vi "CMC温度读取.vi"(8 "error in":errorcluster caption="错误输入", 11 "Channel":u16=81 format="%.0x") -> (0 "error out":errorcluster caption="错误输出", 2 "CMC1温度":i32[](array[numeric]), 3 "CMC2温度":i32[](array[numeric]))   [LabVIEW 2020]
uses:
  <userlib>/PCANBasic/PCANBasic.lvlib
panel:
  out "function return 2":u32 format="%.0x"
  out "function return 3":u32 format="%.0x"
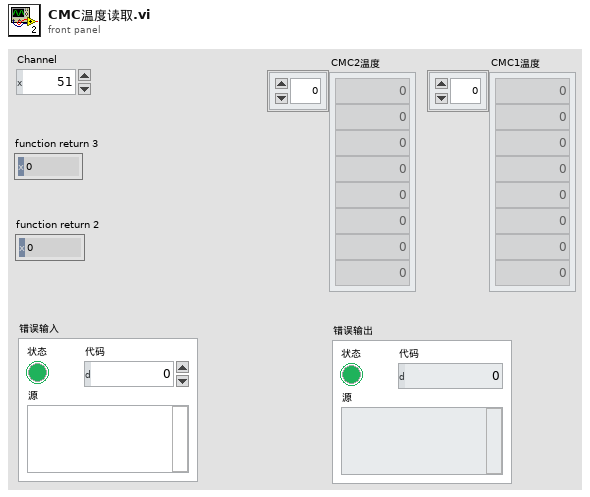
[diagram p1: front panel]
types:
  T1 = typedef "PCANBasic.lvlib/TPCANStatus.ctl" = u32
  T2 = typedef "PCANBasic.lvlib/TPCANMsgFD.ctl" = cluster{"ID":u32, "MSGTYPE":u8, "DLC":u8, "DATA":cluster{"[0]":u8, "[1]":u8, "[2]":u8, "[3]":u8, "[4]":u8, "[5]":u8, "[6]":u8, "[7]":u8, "[8]":u8, "[9]":u8, "[10]":u8, "[11]":u8, "[12]":u8, "[13]":u8, "[14]":u8, "[15]":u8, "[16]":u8, "[17]":u8, "[18]":u8, "[19]":u8, "[20]":u8, "[21]":u8, "[22]":u8, "[23]":u8, "[24]":u8, "[25]":u8, "[26]":u8, "[27]":u8, "[28]":u8, "[29]":u8, "[30]":u8, "[31]":u8, "[32]":u8, "[33]":u8, "[34]":u8, "[35]":u8, "[36]":u8, "[37]":u8, "[38]":u8, "[39]":u8, "[40]":u8, "[41]":u8, "[42]":u8, "[43]":u8, "[44]":u8, "[45]":u8, "[46]":u8, "[47]":u8, "[48]":u8, "[49]":u8, "[50]":u8, "[51]":u8, "[52]":u8, "[53]":u8, "[54]":u8, "[55]":u8, "[56]":u8, "[57]":u8, "[58]":u8, "[59]":u8, "[60]":u8, "[61]":u8, "[62]":u8, "[63]":u8}}
  T3 = cluster{"[0]":u8, "[1]":u8, "[2]":u8, "[3]":u8, "[4]":u8, "[5]":u8, "[6]":u8, "[7]":u8, "[8]":u8, "[9]":u8, "[10]":u8, "[11]":u8, "[12]":u8, "[13]":u8, "[14]":u8, "[15]":u8, "[16]":u8, "[17]":u8, "[18]":u8, "[19]":u8, "[20]":u8, "[21]":u8, "[22]":u8, "[23]":u8, "[24]":u8, "[25]":u8, "[26]":u8, "[27]":u8, "[28]":u8, "[29]":u8, "[30]":u8, "[31]":u8, "[32]":u8, "[33]":u8, "[34]":u8, "[35]":u8, "[36]":u8, "[37]":u8, "[38]":u8, "[39]":u8, "[40]":u8, "[41]":u8, "[42]":u8, "[43]":u8, "[44]":u8, "[45]":u8, "[46]":u8, "[47]":u8, "[48]":u8, "[49]":u8, "[50]":u8, "[51]":u8, "[52]":u8, "[53]":u8, "[54]":u8, "[55]":u8, "[56]":u8, "[57]":u8, "[58]":u8, "[59]":u8, "[60]":u8, "[61]":u8, "[62]":u8, "[63]":u8}
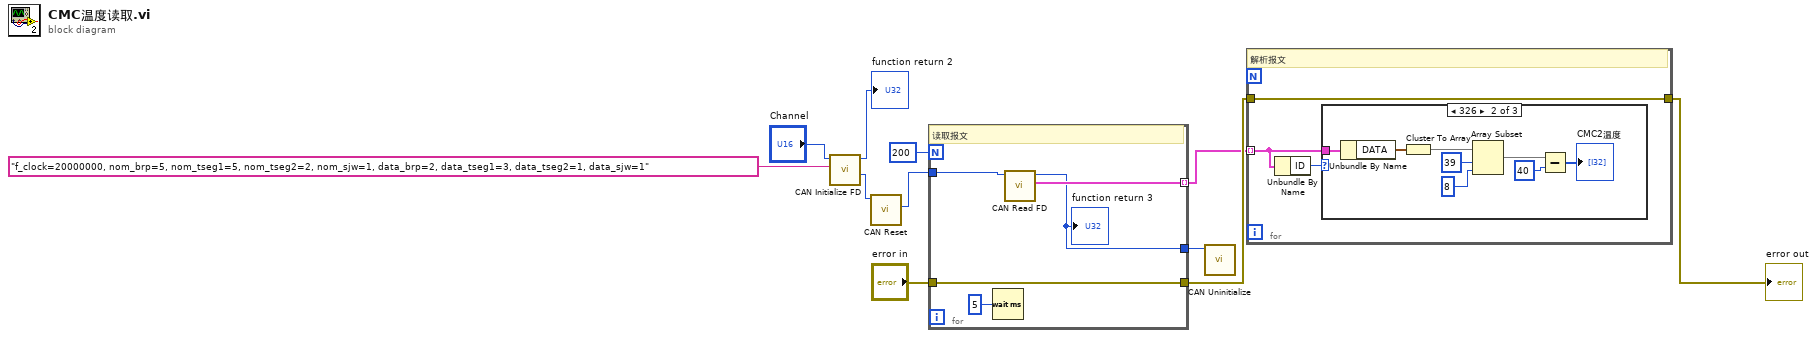
[diagram p0: block diagram]
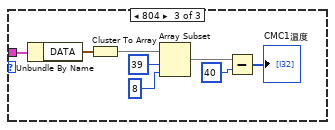
[diagram p3: hidden frame]
diagram:
  n1 = call <userlib>:"CAN Initialize FD.vi"("BitrateFD"="f_clock=20000000, nom_brp=5, nom_tseg1=5, nom_tseg2=2, nom_sjw=1, data_brp=2, data_tseg1=3, data_tseg2=1, data_sjw=1", "Channel"="Channel") -> ("Channel out"=w3:u16, "TCANStatus"=→"function return 2":T1)  [unwired: 6 in, 2 out]
  n2 = call <userlib>:"CAN Reset.vi"("Channel in"=w3) -> ("Channel out"=w2:u16)  [unwired: 8 in, 2 out]
  n3 = for {
    N: 200 -> [_]
    tunnel: [w15] -> w1 mode=indexing
    tunnel: [w14] -> w7
    tunnel: "error in" -> [w13]
    tunnel: [w13] -> w5
    tunnel: w2 -> [w12]
    # "读取报文"
    n4 = Wait (ms)(milliseconds to wait=u32 5 ("等待时间（毫秒）")) -> ()  [unwired: 1 out]
    n5 = call <userlib>:"CAN Read FD.vi"("Channel"=w12) -> ("MessageBuffer out"=w15:T2, "TCANStatus"=w14:T1)  [unwired: 7 in, 2 out]
    "function return 3" <- w14
  }
  n6 = call <userlib>:"CAN Uninitialize.vi"("Channel"=w7) -> ()  [unwired: 9 in, 2 out]
  n7 = for {
    tunnel: w1 -> [w18] mode=indexing
    tunnel: w5 -> [w17]
    tunnel: [w17] -> w4
    # "解析报文"
    n8 = Unbundle By Name(w18) -> ("ID"=w19:u32)
    n9 = case shown="326" w19 {
      tunnel: w18 -> [_ w21 w33]
      frame 0, Default {
      }
      frame 806 {
        n10 = Unbundle By Name(w21) -> ("DATA"=w25:T3)
        n11 = Cluster To Array(cluster=w25) -> (array=w24:u8[])
        n12 = Array Subset(array=w24, index=39 ("索引"), length=8 ("长度")) -> (w20:u8[])
        n13 = Subtract(x=w20, y=40) -> (x-y=→"CMC2温度":i32[])
      }
      frame 804 {
        n14 = Unbundle By Name(w33) -> ("DATA"=w32:T3)
        n15 = Cluster To Array(cluster=w32) -> (array=w31:u8[])
        n16 = Array Subset(array=w31, index=39 ("索引"), length=8 ("长度")) -> (w28:u8[])
        n17 = Subtract(x=w28, y=40) -> (x-y=→"CMC1温度":i32[])
      }
    }
  }
  "error out" <- w4
